vi "Set Output Frequency.vi"(8 "error in (no error)":errorcluster, 10 "Frequency":dbl, 11 "RP Instrument in":refnum<class "RP Instrument.lvclass">) -> (0 "error out":errorcluster, 3 "RP Instrument out":refnum<class "RP Instrument.lvclass">)   [LabVIEW 2015, in "RP Instrument.lvclass"]
uses:
  RP Instrument.lvclass
  RP Command.ctl
  RP Config Offsets.ctl
  RP Instrument.lvclass/RP Instrument.ctl
  RP Communicator/RP Communicator.lvclass
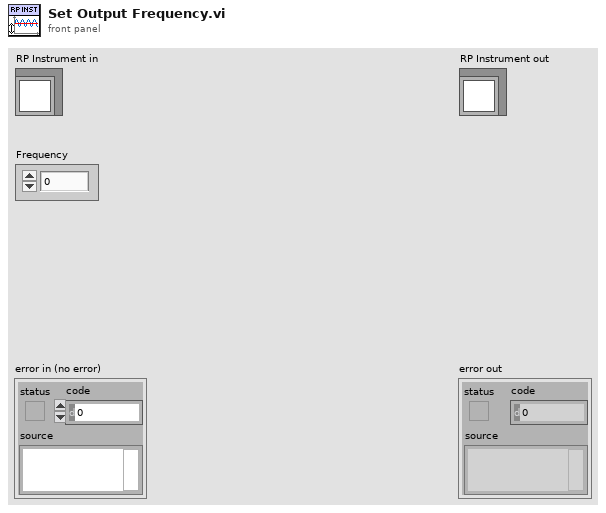
[diagram p1: front panel]
types:
  T1 = typedef "RP Command.ctl" = enum16{"Reset", "Read IDN", "Stop server", "Get status", "Get temperature", "Connect client", "Arm", "Software trigger", "Get whole buffer", "Get chunk", "System call", "Get config", "Set config", "Recieve data", "Play pattern", "Transmit data"}
  T2 = typedef "RP Config Offsets.ctl" = u16
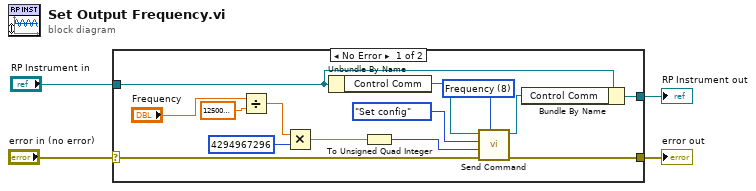
[diagram p0: block diagram]
diagram:
  n1 = case shown="No Error" "error in (no error)" {
    selector: "error in (no error)" -> [w9 w20]
    tunnel: [w8 w20] -> w3
    tunnel: [w7 w19] -> w1
    tunnel: "RP Instrument in" -> [w13 w19]
    frame No Error {
      w5 = T2 8 items=["Config flags"=0, "Record length"=4, "Frequency"=8, "Decimation"=12, "LED"=16, "DDS delay"=28] ("Config offset")
      n2 = Divide(x="Frequency", y=125000000.0) -> (x/y=w16:dbl)
      n3 = Multiply(x=w16, y=i64 4294967296) -> (x*y=w15:dbl)
      n4 = Unbundle By Name(w13) -> ("Control Comm"=w12:refnum<class "RP Communicator.lvclass">)
      n5 = To Unsigned Quad Integer(1:w15) -> (0:w10:u64)
      n6 = call-dynamic "Send Command.vi"("Config offset"=w5, "error in (no error)"=w9, "Command payload"=w10, "Command number"=RP_Command."Set config", "RP Communicator in"=w12) -> ("error out"=w8:errorcluster, "RP Communicator out"=w6:refnum<class "RP Communicator.lvclass">)  [unwired: 5 in]
      n7 = Bundle By Name(cluster=w13, "Control Comm"=w6) -> (w7:refnum<class "RP Instrument.lvclass">)
    }
    frame Error {
    }
  }
  "error out" <- w3
  "RP Instrument out" <- w1
